vi "IsCollision.vi"(1 "Segment B":T1, 2 "Collisions":T2[](array[typedef])) -> (0 "Collision?":bool)   [LabVIEW 2015, in "Level.lvclass"]
uses:
  Level.lvclass
  Segment.ctl
  Point.ctl
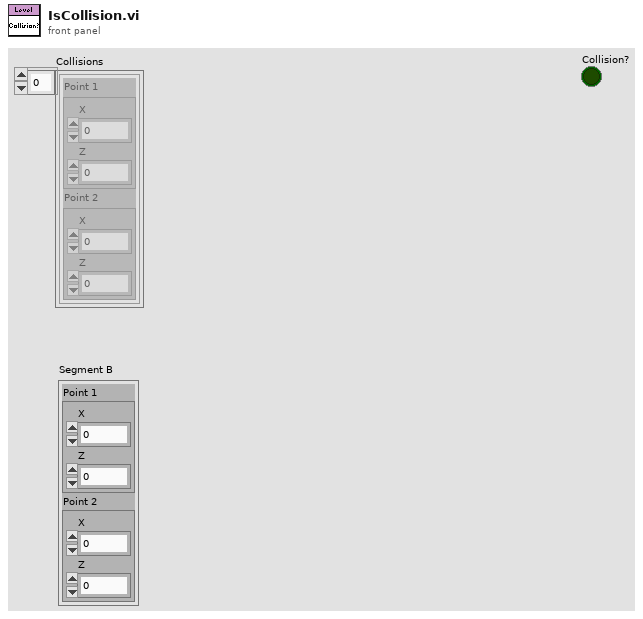
[diagram p1: front panel]
types:
  T1 = cluster{"Point 1":cluster{"Z":dbl, "X":dbl}, "Point 2":cluster{"Z":dbl, "X":dbl}}
  T2 = typedef "Level.lvclass/Segment.ctl" = cluster{"Point 1":T3, "Point 2":T3}
  T3 = typedef "Level.lvclass/Point.ctl" = cluster{"Z":dbl, "X":dbl}
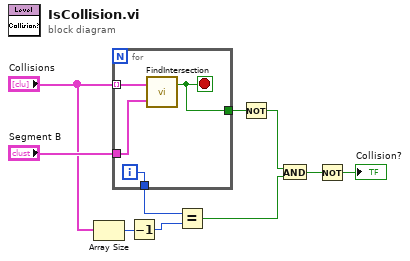
[diagram p0: block diagram]
diagram:
  n1 = Array Size(array="Collisions") -> (size(s)=w4:i32)
  n2 = for {
    tunnel: "Collisions" -> [w14] mode=indexing
    tunnel: "Segment B" -> [w13]
    tunnel: [w12] -> w8
    tunnel: [w11] -> w5
    i -> [w11]
    stop <- w12 stop-if-true
    n3 = call "FindIntersection.vi"("Segment B"=w13, "Segment A"=w14) -> ("Segments Intersect?"=w12:bool)  [unwired: 1 out]
  }
  n4 = Decrement(x=w4) -> (x-1=w3:i32)
  n5 = Equal?(x=w5, y=w3) -> (x = y?=w6:bool)
  n6 = Not(x=w8) -> (.not. x?=w7:bool)
  n7 = And(x=w7, y=w6) -> (x .and. y?=w2:bool)
  n8 = Not(x=w2) -> (.not. x?=→"Collision?":bool)
